vi "myRIO_BRig_RT_dataLick_iState__atLick.vi"() -> (2 "output_iState__atLick":i32)   [LabVIEW 2014]
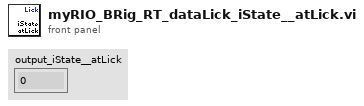
[diagram p1: front panel]
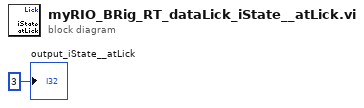
[diagram p0: block diagram]
diagram:
  "output_iState__atLick" <- 3 ("output_iBlock")
